vi "Delete.vi"(8 "error in (no error)":errorcluster, 10 "Path":string, 11 "FTP in":refnum<class "FTP.lvclass">) -> (0 "error out":errorcluster, 3 "FTP out":refnum<class "FTP.lvclass">)   [LabVIEW 2016, in "RT Management.lvlib" / "FTP.lvclass"]
uses:
  FTP.lvclass
  FTP.lvclass/FTP.ctl
  Get Session.vi
  <vilib>/FTP/NI_FTP.lvlib
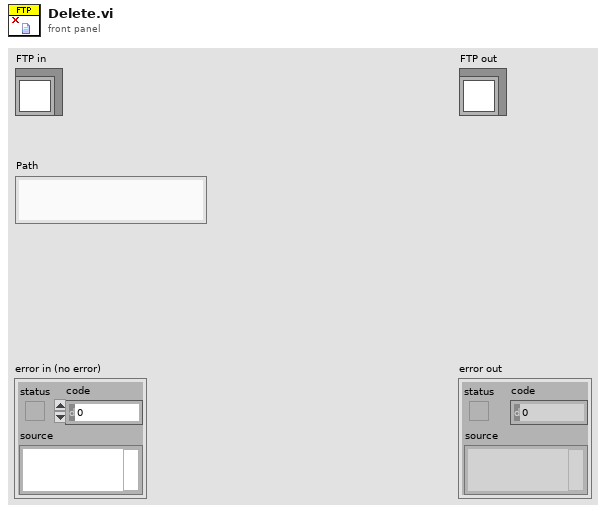
[diagram p1: front panel]
types:
  T1 = typedef "RT Management.lvlib/File Transfer Behavior.lvclass/Type.ctl" = enum16{"unknown", "file", "directory"}
  T2 = typedef "NI_FTP.lvlib/FTP Session.ctl" = refnum<k5>
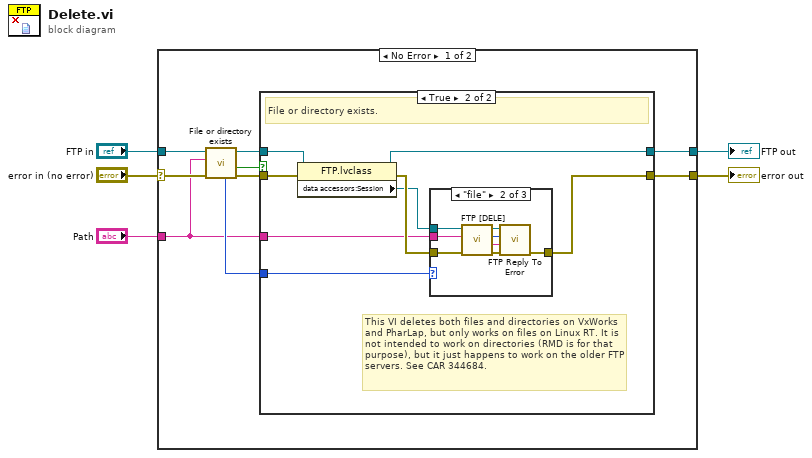
[diagram p0: block diagram]
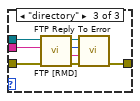
[diagram p4: hidden frame]
diagram:
  n1 = case shown="No Error" "error in (no error)" {
    selector: "error in (no error)" -> [w14 w43]
    tunnel: "FTP in" -> [w13 w42]
    tunnel: [w10 w42] -> w3
    tunnel: [w8 w43] -> w2
    tunnel: "Path" -> [w7 _]
    frame No Error {
      n2 = call-dynamic "File or directory exists.vi"("error in (no error)"=w14, "Path"=w7, "FTP in"=w13) -> ("error out"=w12:errorcluster, "Exists?"=w6:bool, "FTP out"=w11:refnum<class "FTP.lvclass">, "Type"=w9:T1)  [unwired: 4 in, 1 out]
      n3 = case shown="True" w6 {
        tunnel: w12 -> [w15 w24]
        tunnel: w11 -> [w16 w23]
        tunnel: [w16 w22] -> w10
        tunnel: w9 -> [_ w21]
        tunnel: [w15 w18] -> w8
        tunnel: w7 -> [_ w17]
        frame False {
          # "Nothing exists at the path."
        }
        frame True {
          # "This VI deletes both files and directories on VxWorks and PharLap, but only works on files on Linux RT. It is not intended to work on directories (RMD is for that purpose), but it just happens to work on the older FTP servers. See CAR 344684."
          # "File or directory exists."
          n4 = property class="FTP.lvclass"(reference=w23, error in=w24) -> (reference out=w22:refnum<class "FTP.lvclass">, error out=w20:errorcluster, "data accessors:Session"=w19:T2)
          n5 = case shown="\"file\"" w21 {
            tunnel: w20 -> [w25 w32 w39]
            tunnel: w19 -> [_ w31 w35]
            tunnel: [w25 w30 w41] -> w18
            tunnel: w17 -> [_ w26 w34]
            frame "unknown" {
            }
            frame "file" {
              n6 = call <vilib>:"FTP [DELE].vi"("error in (no error)"=w32, "file path"=w26, "ftp session"=w31) -> ("error out"=w33:errorcluster, "reply string"=w27:string, "reply code"=w28:i32, "ftp session out"=w29:T2)  [unwired: 5 in]
              n7 = call <vilib>:"FTP Reply To Error.vi"("error in (no error)"=w33, "reply string in"=w27, "reply code in"=w28, "ftp session"=w29) -> ("error out"=w30:errorcluster)  [unwired: 3 out]
            }
            frame "directory" {
              n8 = call <vilib>:"FTP [RMD].vi"("error in (no error)"=w39, "directory path"=w34, "ftp session"=w35) -> ("error out"=w40:errorcluster, "reply string"=w38:string, "reply code"=w37:i32, "ftp session out"=w36:T2)  [unwired: 5 in]
              n9 = call <vilib>:"FTP Reply To Error.vi"("error in (no error)"=w40, "reply string in"=w38, "reply code in"=w37, "ftp session"=w36) -> ("error out"=w41:errorcluster)  [unwired: 3 out]
            }
          }
        }
      }
    }
    frame Error {
    }
  }
  "error out" <- w2
  "FTP out" <- w3
